vi "testCalcul_CdG.vi"() -> ()   [LabVIEW 2020]
uses:
  <vilib>/Analysis/baseanly.llb/Mean (DBL).vi
  <vilib>/Analysis/NI_AALBase.lvlib
panel:
  out "CdGOut [Pixels]":dbl[](array[numeric])
  out "mean":dbl format="%g"
  out "Waveform Graph":dbl[](graph)
  in  "imagette_1":i16[][](array[numeric])
  in  "imagette_0":i16[][](array[numeric])
  in  "CdG in":dbl[](array[numeric])=[99.0, 100.0, 1000.0, 2000.0]
  out "error out":errorcluster
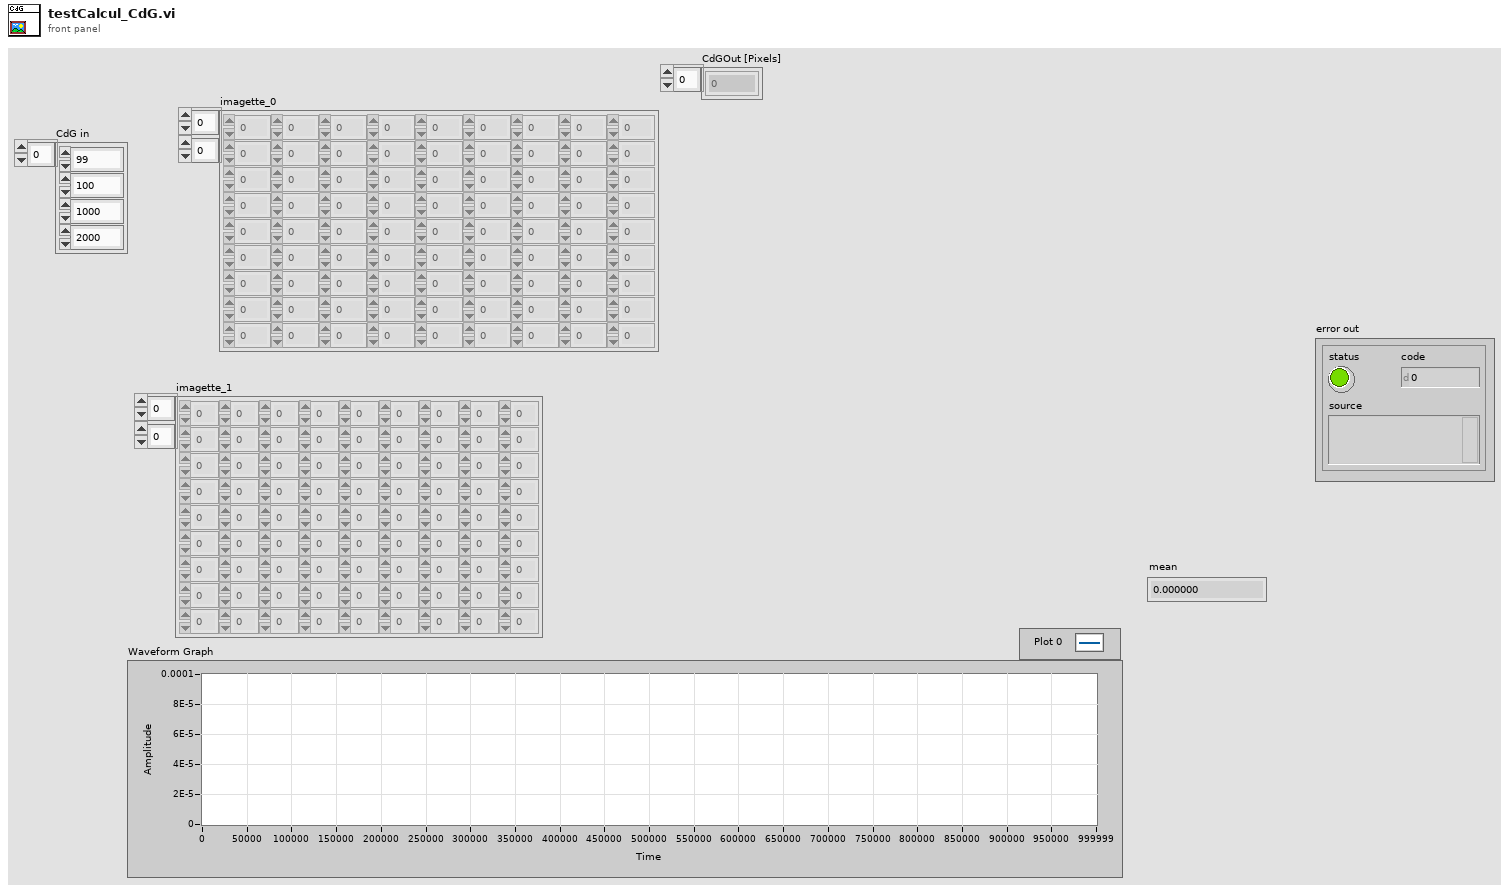
[diagram p1: front panel]
types:
  T1 = enum16{"Initialisation", "Calcul CdG a", "Calcul CdG b"}
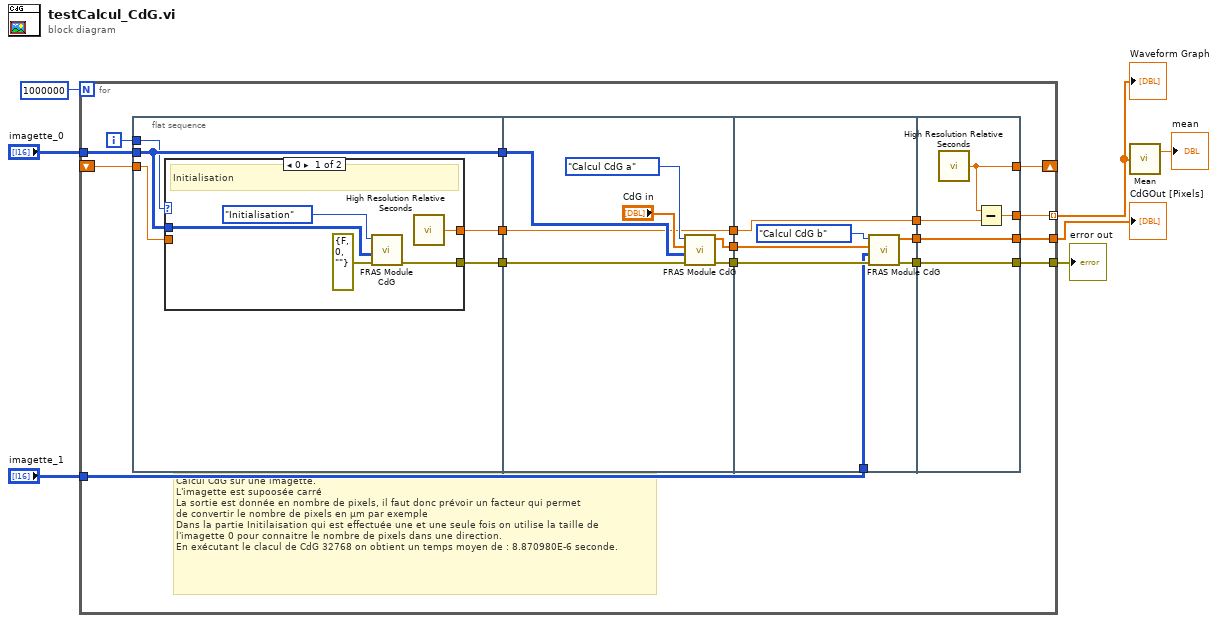
[diagram p0: block diagram]
diagram:
  n1 = for {
    N: 1000000 -> [_]
    tunnel: "imagette_0" -> [w20]
    tunnel: "imagette_1" -> [w19]
    shift-right: [w14] -> _
    shift-left: _ -> [w13]
    tunnel: [w12] -> w4 mode=indexing
    tunnel: [w10] -> w2
    tunnel: [w8] -> w1
    i -> [w18]
    # "Calcul CdG sur une imagette. \nL'imagette est supoosée carré \nLa sortie est donnée en nombre de pixels, il faut donc prévoir un facteur qui permet \nde convertir le nombre de pixels en µm par exemple\nDans la partie Initilaisation qui est effectuée une et une seule fois on utilise la taille de \nl'imagette 0 pour connaitre le nombre de pixels dans une direction.\nEn exécutant le clacul de CdG 32768 on obtient un temps moyen de : 8.870980E-6 seconde."
    n2 = flat-sequence {
      tunnel: w20 -> [w29]
      tunnel: [w28] -> w24
      tunnel: [w29] -> w23
      tunnel: w18 -> [w27]
      tunnel: [w26] -> w17
      tunnel: w13 -> [w25]
      tunnel: w24 -> [w40]
      tunnel: w23 -> [w37]
      tunnel: [w42] -> w22
      tunnel: [w38] -> w21
      tunnel: w17 -> [w36]
      tunnel: [w36] -> w16
      tunnel: w22 -> [w49]
      tunnel: w21 -> [w47]
      tunnel: w19 -> [w48]
      tunnel: w16 -> [w45]
      tunnel: [w45] -> w15
      tunnel: [w44] -> w11
      tunnel: [w43] -> w9
      tunnel: w15 -> [w53]
      tunnel: [w54] -> w14
      tunnel: [w52] -> w12
      tunnel: [w51] -> w10
      tunnel: w11 -> [w51]
      tunnel: w9 -> [w50]
      tunnel: [w50] -> w8
      frame #0 {
        n3 = case shown="0" w27 {
          tunnel: w29 -> [w30 _]
          tunnel: [w32 _] -> w28
          tunnel: [w31 w35] -> w26
          tunnel: w25 -> [_ w35]
          frame 0 {
            # "Initialisation"
            n4 = call "FRAS Module CdG.vi"("error in"=errorcluster {"status"=FALSE, "code"=0, "source"=""}, "Imagette seuillée"=w30, "Mode CdG"=T1."Initialisation") -> ("error out"=w32:errorcluster)  [unwired: 6 in, 1 out]
            n5 = call <vilib>:"High Resolution Relative Seconds.vi"() -> ("relative seconds"=w31:dbl)
          }
          frame 1, Default {
            # "VOID"
          }
        }
      }
      frame #1 {
        n6 = call "FRAS Module CdG.vi"("error in"=w40, "Imagette seuillée"=w37, "inCdG[Pixels]"="CdG in", "Mode CdG"=T1."Calcul CdG a") -> ("error out"=w42:errorcluster, "CdGOut [Pixels]"=w38:dbl[])  [unwired: 5 in]
      }
      frame #2 {
        n7 = call "FRAS Module CdG.vi"("error in"=w49, "Imagette seuillée"=w48, "inCdG[Pixels]"=w47, "Mode CdG"=T1."Calcul CdG b") -> ("error out"=w43:errorcluster, "CdGOut [Pixels]"=w44:dbl[])  [unwired: 5 in]
      }
      frame #3 {
        n8 = call <vilib>:"High Resolution Relative Seconds.vi"() -> ("relative seconds"=w54:dbl)
        n9 = Subtract(x=w54, y=w53) -> (x-y=w52:dbl)
      }
    }
  }
  "Waveform Graph" <- w4
  "CdGOut [Pixels]" <- w2
  "error out" <- w1
  n10 = call-poly <vilib>:"Mean.vi"("X"=w4) -> ("mean"=→"mean":dbl)  [unwired: 1 out]
